vi "Initialize.vi"(8 "error in (no error)":errorcluster, 11 "Ismatech Settings":T1={"VISA resource name"="", "Simulated?"=FALSE, "Pump Number"=1.0, "Reverse?"=FALSE} {"Pump Number" min=1.0 max=20.0 step=1.0}) -> (0 "error out":errorcluster, 1 "Initialized":bool, 2 "No Pump Connected":bool=TRUE, 3 "Ismatech Settings":T1={"VISA resource name"="", "Simulated?"=FALSE, "Pump Number"=1.0, "Reverse?"=FALSE} {"Pump Number" min=1.0 max=20.0 step=1.0})   [LabVIEW 2021, in "Ismatec ISM 831C.lvlib"]
uses:
  Ismatec ISM 831C.lvlib
  Controls/Ismatech ISM831C Settings Cluster.ctl
  <vilib>/Instr/_visa.llb/VISA Configure Serial Port (Instr).vi
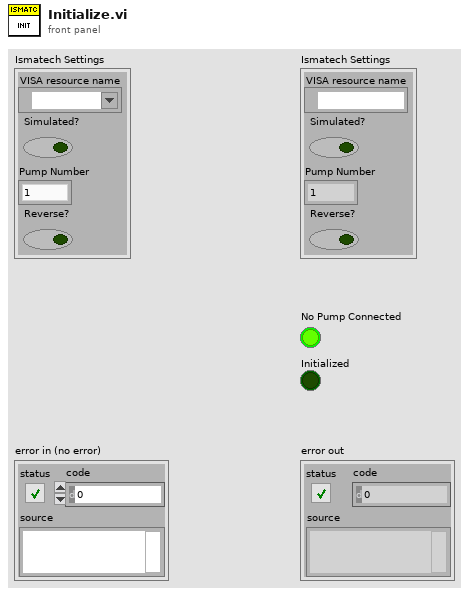
[diagram p1: front panel]
types:
  T1 = typedef "Ismatec ISM 831C.lvlib/Ismatech ISM831C Settings Cluster.ctl" = cluster{"VISA resource name":refnum<visa-resource-name>, "Simulated?":bool, "Pump Number":dbl, "Reverse?":bool}
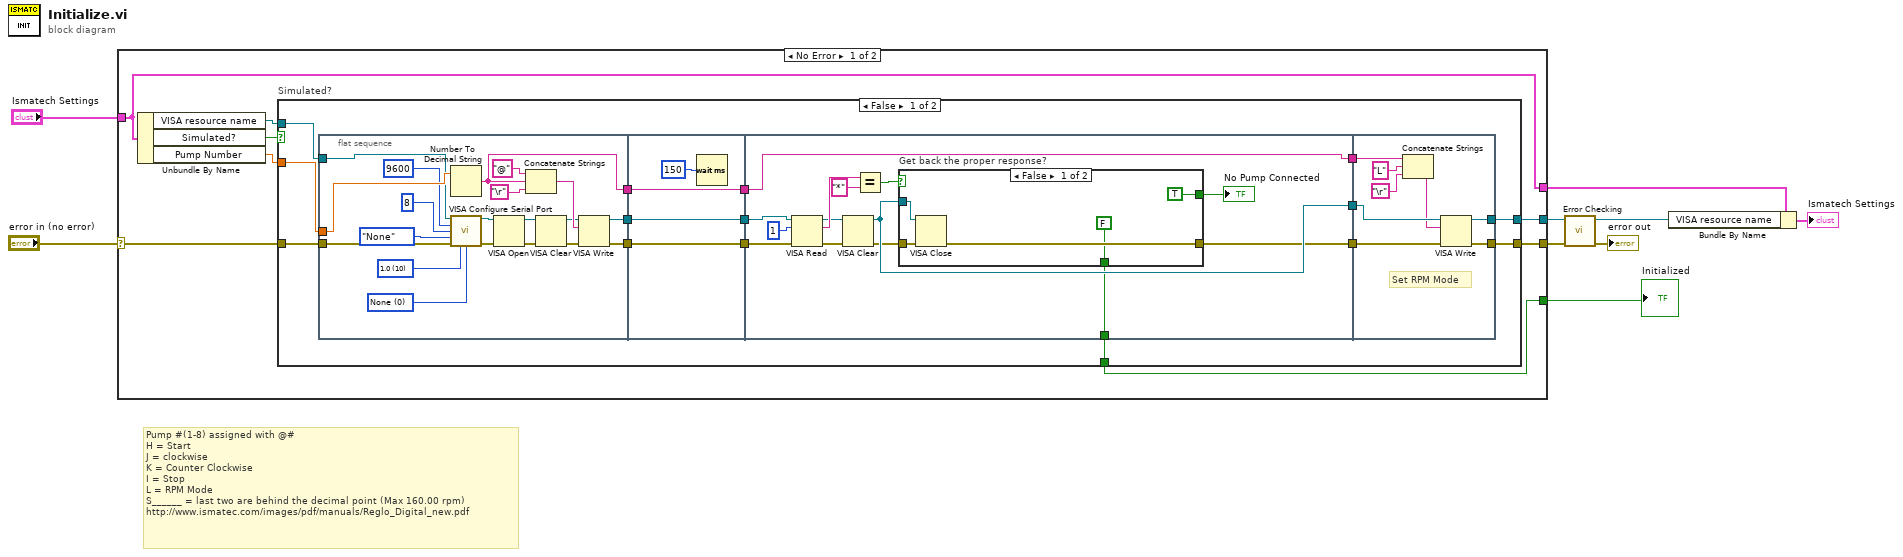
[diagram p0: block diagram]
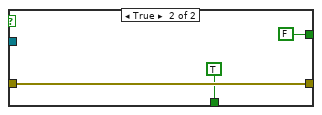
[diagram p2: hidden frame]
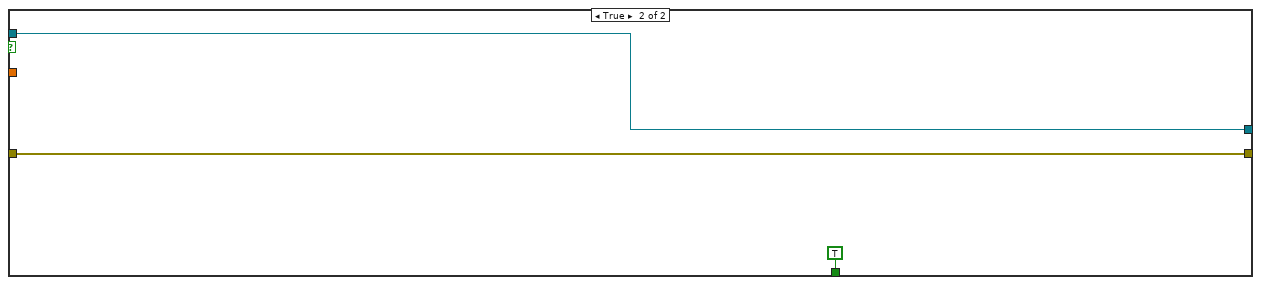
[diagram p3: hidden frame]
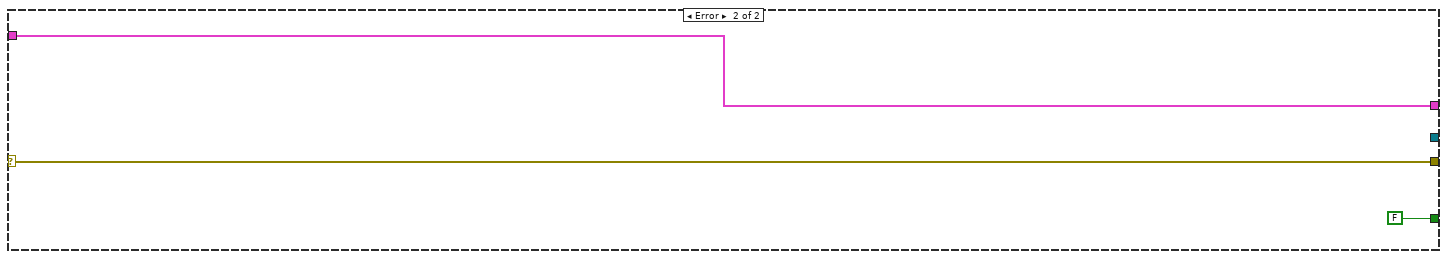
[diagram p4: hidden frame]
diagram:
  # "Pump #(1-8) assigned with @#\nH = Start\nJ = clockwise\nK = Counter Clockwise\nI = Stop\nL = RPM Mode\nS______ = last two are behind the decimal point (Max 160.00 rpm)\nhttp://www.ismatec.com/images/pdf/manuals/Reglo_Digital_new.pdf"
  n1 = case shown="No Error" "error in (no error)" {
    selector: "error in (no error)" -> [w13 w92]
    tunnel: "Ismatech Settings" -> [w12 w91]
    tunnel: [w16 w92] -> w4
    tunnel: [w12 w91] -> w3
    tunnel: [w11 _] -> w2
    tunnel: [w10 FALSE] -> w1
    frame No Error {
      n2 = Unbundle By Name(w12) -> ("VISA resource name"=w14:refnum<visa-resource-name>, "Simulated?"=w17:bool, "Pump Number"=w15:dbl)
      n3 = case "Simulated?" shown="False" w17 {
        tunnel: [w32 w88] -> w16
        tunnel: [w31 w89] -> w11
        tunnel: w15 -> [w30 _]
        tunnel: w14 -> [w29 w89]
        tunnel: w13 -> [w28 w88]
        tunnel: [w18 TRUE] -> w10
        frame False {
          n4 = flat-sequence {
            tunnel: w30 -> [w50]
            tunnel: w29 -> [w47]
            tunnel: w28 -> [w43]
            tunnel: [w40] -> w26
            tunnel: [w38] -> w25
            tunnel: [w33] -> w21
            tunnel: [w55] -> w27
            tunnel: w26 -> [w55]
            tunnel: w25 -> [w54]
            tunnel: [w54] -> w24
            tunnel: w21 -> [w53]
            tunnel: [w53] -> w20
            tunnel: w27 -> [w69]
            tunnel: w24 -> [w68]
            tunnel: [w61] -> w23
            tunnel: [w63] -> w22
            tunnel: w20 -> [w59]
            tunnel: [w59] -> w19
            tunnel: [w57] -> w18
            tunnel: [w85] -> w31
            tunnel: [w83] -> w32
            tunnel: w23 -> [w84]
            tunnel: w22 -> [w86]
            tunnel: w19 -> [w82]
            frame #0 {
              w41 = u16 0 items=["None", "XON/XOFF", "RTS/CTS", "XON/XOFF & RTS/CTS", "DTR/DSR", "XON/XOFF & DTR/DSR"] ("flow control (0:none)")
              w42 = u16 10 items=["1.0"=10, "1.5"=15, "2.0"=20] ("stop bits (10: 1 bit)")
              n5 = Number To Decimal String(number=w50) -> (decimal integer string=w33:string)  [unwired: 1 in]
              n6 = call-poly "VISA Configure Serial Port"("VISA resource name"=w47, "baud rate (9600)"=u32 9600, "data bits (8)"=u16 8, "parity (0:none)"=enum16{"None", "Odd", "Even", "Mark", "Space"}."None", "error in (no error)"=w43, "stop bits (10: 1 bit)"=w42, "flow control (0:none)"=w41) -> ("VISA resource name out"=w52:refnum<visa-resource-name>, "error out"=w51:errorcluster)  [unwired: 7 in]
              n7 = VISA Open(error in (no error)=w51, VISA resource name=w52) -> (VISA resource name=w37:refnum<visa-resource-name>, error out=w36:errorcluster)  [unwired: 3 in]
              n8 = Concatenate Strings("@" ("string"), w33, "\r") -> (w39:string)
              n9 = VISA Clear(VISA resource name=w37, error in (no error)=w36) -> (VISA resource name out=w35:refnum<visa-resource-name>, error out=w34:errorcluster)
              n10 = VISA Write(VISA resource name=w35, write buffer=w39, error in (no error)=w34) -> (VISA resource name out=w40:refnum<visa-resource-name>, error out=w38:errorcluster)  [unwired: 1 out]
            }
            frame #1 {
              n11 = Wait (ms)(milliseconds to wait=u32 150) -> ()  [unwired: 1 out]
            }
            frame #2 {
              n12 = VISA Read(VISA resource name=w69, byte count=u32 1, error in (no error)=w68) -> (VISA resource name out=w64:refnum<visa-resource-name>, read buffer=w67:string, error out=w65:errorcluster)  [unwired: 1 out]
              n13 = VISA Clear(VISA resource name=w64, error in (no error)=w65) -> (VISA resource name out=w63:refnum<visa-resource-name>, error out=w60:errorcluster)
              n14 = Equal?(x=w67, y="*") -> (x = y?=w62:bool)
              n15 = case "Get back the proper response?" shown="False" w62 {
                tunnel: w63 -> [w75 _]
                tunnel: w60 -> [w74 w78]
                tunnel: [w73 w78] -> w61
                tunnel: [TRUE FALSE] -> w58
                tunnel: [FALSE TRUE] -> w57
                frame False {
                  n16 = VISA Close(VISA resource name=w75, error in (no error)=w74) -> (error out=w73:errorcluster)
                }
                frame True {
                }
              }
              "No Pump Connected" <- w58
            }
            frame #3 {
              # "Set RPM Mode"
              n17 = Concatenate Strings(w82, "L" ("string"), "\r") -> (w79:string)
              n18 = VISA Write(VISA resource name=w86, write buffer=w79, error in (no error)=w84) -> (VISA resource name out=w85:refnum<visa-resource-name>, error out=w83:errorcluster)  [unwired: 1 out]
            }
          }
        }
        frame True {
        }
      }
    }
    frame Error {
    }
  }
  "Initialized" <- w1
  n19 = call "Error Checking.vi"("error in (no error)"=w4, "VISA resource name"=w2) -> ("error out"=→"error out":errorcluster, "VISA resource name"=w7:refnum<visa-resource-name>)  [unwired: 7 in, 1 out]
  n20 = Bundle By Name(cluster=w3, "VISA resource name"=w7) -> (→"Ismatech Settings":T1)
